vi "acquireWhenStop.vi"() -> ()   [LabVIEW 2016]
uses:
  <vilib>/Utility/file.llb/Write Delimited Spreadsheet (DBL).vi
panel:
  out "即将记录":dbl=1.0
  out "osc stoped":bool
  in  "OSC in":refnum<visa-resource-name>
  in  "start":bool
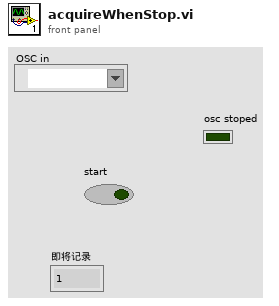
[diagram p1: front panel]
types:
  T1 = typedef "NI_Matrix.lvlib/RealMatrix.ctl" = dbl[][]
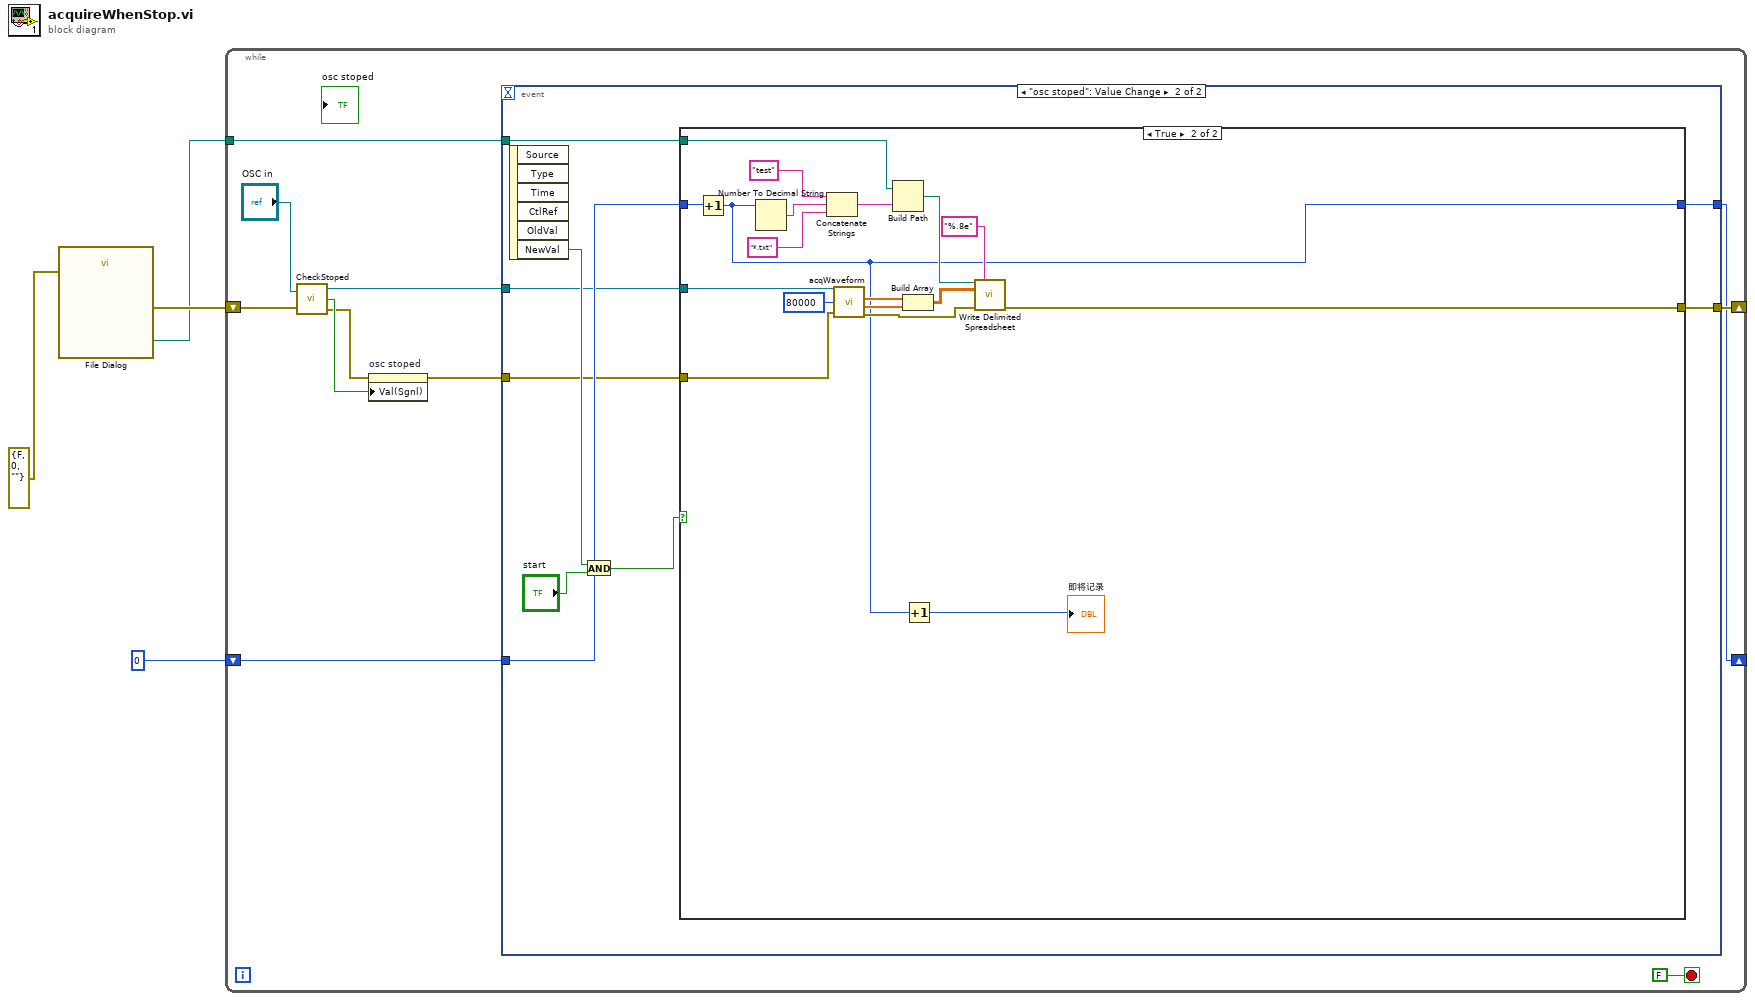
[diagram p0: block diagram]
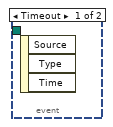
[diagram p2: hidden frame]
diagram:
  n1 = call "File Dialog"("error in"=errorcluster {"status"=FALSE, "code"=0, "source"=""} ("error in (no error)")) -> ("selected path"=w1:path, "error out"=w2:errorcluster)  [unwired: 11 in, 2 out]
  n2 = while {
    tunnel: w1 -> [w7]
    shift-right: [w6] -> _
    shift-left: w2 -> [w14]
    shift-right: [w5] -> _
    shift-left: 0 -> [w10]
    stop <- FALSE stop-if-true
    n3 = call "CheckStoped.vi"("OSC in"="OSC in", "error in (no error)"=w14) -> ("OSC out"=w9:refnum<visa-resource-name>, "Stopped?"=w12:bool, "error out"=w11:errorcluster)
    n4 = property on="osc stoped" class="Bool (strict)"(error in=w11, "Val(Sgnl)"=w12) -> (error out=w8:errorcluster)  [unwired: 1 in, 1 out]
    n5 = event shown="[1] \"osc stoped\": Value Change" {
      selector: _ -> [_ _]
      dyn-events: _ -> [_ _]
      timeout: _ -> [_ _]
      tunnel: w10 -> [_ w21]
      tunnel: w9 -> [_ w20]
      tunnel: w8 -> [_ w19]
      tunnel: w7 -> [_ w18]
      tunnel: [_ w17] -> w6
      tunnel: [_ w16] -> w5
      event Timeout {
        n6 = event-data() -> ()  [unwired: 1 in, 3 out]
      }
      event "osc stoped": Value Change {
        n7 = event-data() -> ("NewVal"=w23:bool)  [unwired: 1 in, 5 out]
        n8 = And(x=w23, y="start") -> (x .and. y?=w22:bool)
        n9 = case shown="True" w22 {
          tunnel: w21 -> [w25 w44]
          tunnel: w20 -> [_ w43]
          tunnel: w19 -> [w26 w41]
          tunnel: w18 -> [_ w33]
          tunnel: [w26 w29] -> w17
          tunnel: [w25 w27] -> w16
          frame False {
          }
          frame True {
            n10 = Increment(x=w44) -> (x+1=w27:i32)
            n11 = Number To Decimal String(number=w27) -> (decimal integer string=w37:string)  [unwired: 1 in]
            n12 = Concatenate Strings("test" ("string"), w37, "*.txt" ("string")) -> (w34:string)
            n13 = call "acqWaveform.vi"("OSC in"=w43, "Points"=u32 80000, "error in (no error)"=w41) -> ("time sequence"=w40:dbl[], "Voltage sequence"=w39:dbl[], "error out"=w30:errorcluster)  [unwired: 1 out]
            n14 = Build Path(base path=w33, name or relative path=w34) -> (appended path=w32:path)
            n15 = Build Array(w40, w39) -> (w38:T1)
            n16 = Increment(x=w27) -> (x+1=→"即将记录":i32)
            n17 = call-poly <vilib>:"Write Delimited Spreadsheet.vi"("file path (dialog if empty)"=w32, "format (%.3f)"="%.8e", "2D data"=w38, "error in (no error)"=w30) -> ("error out"=w29:errorcluster)  [unwired: 10 in, 1 out]
          }
        }
      }
    }
  }
